vi "Reorder Commands.vi"(11 "Array in":T1[](array[typedef])) -> (3 "Array out":T1[](array[typedef]))   [LabVIEW 2020, in "CSM-ScheduledCmdWindow.lvlib"]
uses:
  CSM-ScheduledCmdWindow.lvlib
  Command Timer Item.ctl
  <userlib>/_Hooovahh/Array VIMs/Controls/Enum - Order Ascending Descending.ctl
  a44d329b-48aa-4752-86cb-e8a498e564a4.vi
  8444be56-9229-45c4-8f2e-bfc49e235e73.vi
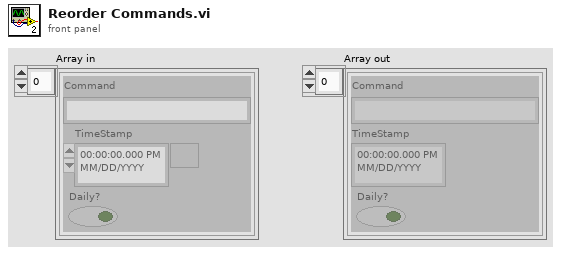
[diagram p1: front panel]
types:
  T1 = typedef "CSM-ScheduledCmdWindow.lvlib/Command Timer Item.ctl" = cluster{"Command":string, "TimeStamp":timestamp, "Daily?":bool}
  T2 = typedef "Enum - Order Ascending Descending.ctl" = enum16{"Ascending", "Descending"}
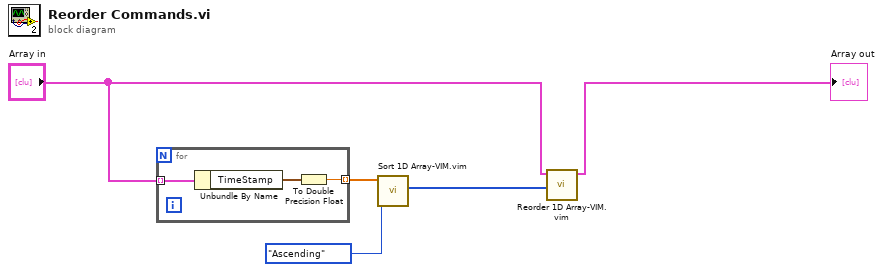
[diagram p0: block diagram]
diagram:
  n1 = for {
    tunnel: "Array in" -> [w8] mode=indexing
    tunnel: [w6] -> w2 mode=indexing
    n2 = Unbundle By Name(w8) -> ("TimeStamp"=w7:timestamp)
    n3 = To Double Precision Float(number=w7) -> (double precision float=w6:dbl)
  }
  n4 = call "Sort 1D Array-VIM.vim"("Order (Ascending)"=Enum_-_Order_Ascending_Descending."Ascending", "Array in"=w2) -> ("Sorted Pointers"=w3:i32[])  [unwired: 8 in, 1 out]
  n5 = call "Reorder 1D Array-VIM.vim"("indices"=w3, "array"="Array in") -> ("reordered array"=→"Array out":T1[])  [unwired: 9 in]
